vi "Calculate Xn-Xn-1.vi"(9 "Point":i32=1, 11 "X":dbl[](array[numeric])) -> (1 "Point":i32, 3 "Xn-Xn-1":dbl[](array[numeric]))   [LabVIEW 2021]
doc: "技术Xn-Xn-m；\nm= Point\n2015-05-27 14:37:52\n蒋松\njiangsong@outlook.com"
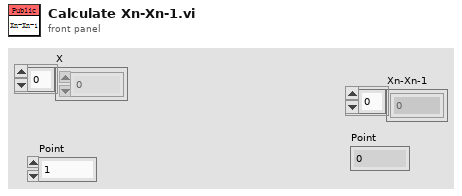
[diagram p1: front panel]
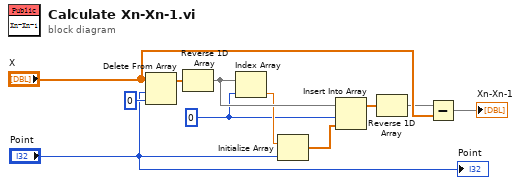
[diagram p0: block diagram]
diagram:
  w1 = 0 ("index")
  n1 = Delete From Array(array="X", length="Point", index=0) -> (array with subset deleted=w9:dbl[])  [unwired: 1 out]
  n2 = Reverse 1D Array(array=w9) -> (reversed array=w8:dbl[])
  n3 = Index Array(array=w8, index=w1) -> (element=w5:dbl)
  n4 = Initialize Array(w5, "Point") -> (w4:dbl[])
  n5 = Insert Into Array(array=w8, index=w1, new element=w4) -> (w7:dbl[])
  n6 = Reverse 1D Array(array=w7) -> (reversed array=w3:dbl[])
  n7 = Subtract(x=w3, y="X") -> (x-y=→"Xn-Xn-1":dbl[])
  "Point" <- "Point"
